vi "FGV Modbus.vi"(6 "Aktion":T1) -> (0 "error out":errorcluster)   [LabVIEW 2020, in "ABB-EL3000.lvlib" / "PMA.lvlib"]
uses:
  PMA.lvlib
  Allgemeine VI/Aktion FGV Modbus.ctl
  Aktion Adressen.ctl
  Allgemeine VI/Aktion Modbus lesen.ctl
  Aktion FGV Messwerte.ctl
  Allgemeine VI/Allgemeine VI.lvlib
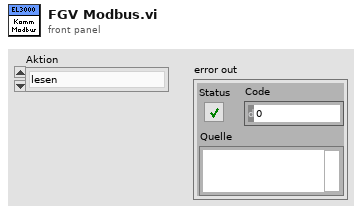
[diagram p1: front panel]
types:
  T1 = typedef "ABB-EL3000.lvlib/Allgemeine VI.lvlib/Aktion FGV Modbus.ctl" = enum16{"lesen", "Verbindung herstellen", "Verbindung trennen", "Komm", "Inaktiv"}
  T2 = typedef "ABB-EL3000.lvlib/PMA.lvlib/Aktion Adressen.ctl" = enum16{"lesen", "initialisieren"}
  T3 = typedef "ABB-EL3000.lvlib/PMA.lvlib/Aktion FGV Messwerte.ctl" = enum16{"lesen", "Messwerte", "Messbereich", "Status", "Diagnose Werte"}
  T4 = typedef "ABB-EL3000.lvlib/Allgemeine VI.lvlib/Aktion Modbus lesen.ctl" = enum16{"Coils", "Discrete Inputs", "Input Register", "Holding Register"}
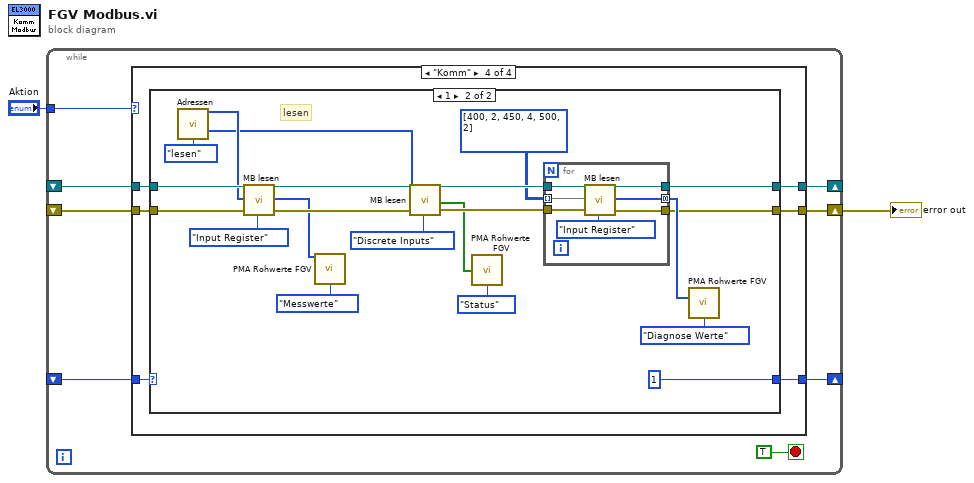
[diagram p0: block diagram]
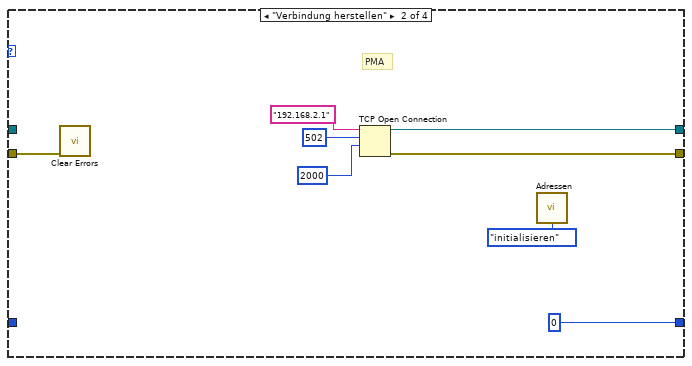
[diagram p3: hidden frame]
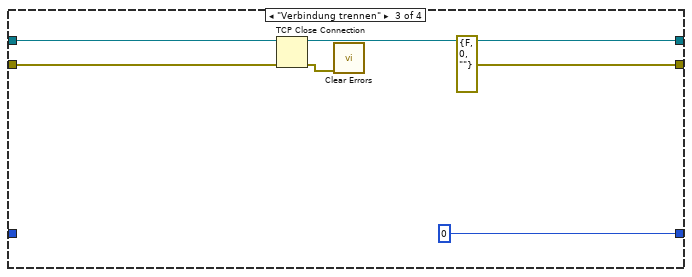
[diagram p4: hidden frame]
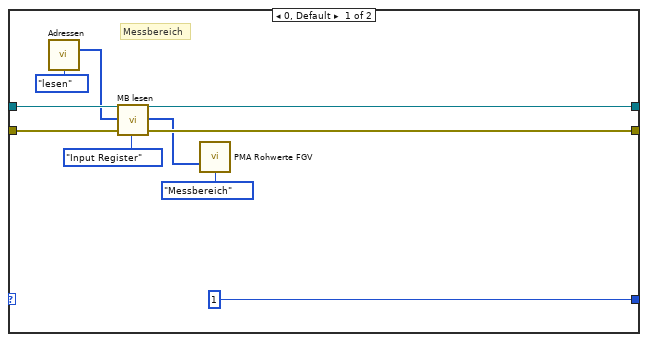
[diagram p5: hidden frame]
diagram:
  n1 = while {
    tunnel: "Aktion" -> [w9]
    shift-right: [w8] -> _
    shift-left: _ -> [w7]
    shift-right: [w6] -> w1
    shift-left: _ -> [w5]
    shift-right: [w3] -> _
    shift-left: _ -> [w4]
    stop <- TRUE stop-if-true
    n2 = case shown="\"Komm\"" w9 {
      tunnel: [w13 w20 w25 w32] -> w8
      tunnel: w7 -> [w13 _ w27 w33]
      tunnel: [w12 w19 errorcluster {"status"=FALSE, "code"=0, "source"=""} ("error out") w30] -> w6
      tunnel: w5 -> [w12 w18 w26 w31]
      tunnel: w4 -> [w11 _ _ w29]
      tunnel: [w11 0 0 w28] -> w3
      frame "lesen", Default {
      }
      frame "Verbindung herstellen" {
        # "PMA"
        n3 = call <vilib>:"Clear Errors.vi"("error in (no error)"=w18) -> ()  [unwired: 5 in, 2 out]
        n4 = TCP Open Connection(address="192.168.2.1" ("Adresse"), remote port or service name=u16 502 ("Netzwerk-Port oder -Dienst"), timeout ms (60000)=2000 ("Timeout in ms (60000)")) -> (connection ID=w20:refnum<k5>, error out=w19:errorcluster)  [unwired: 2 in]
        n5 = call "Adressen.vi"("Aktion"=Aktion_Adressen."initialisieren") -> ()  [unwired: 11 in, 4 out]
      }
      frame "Verbindung trennen" {
        n6 = TCP Close Connection(connection ID=w27, error in (no error)=w26) -> (connection ID out=w25:refnum<k5>, error out=w23:errorcluster)  [unwired: 1 in]
        n7 = call <vilib>:"Clear Errors.vi"("error in (no error)"=w23) -> ()  [unwired: 5 in, 2 out]
      }
      frame "Komm" {
        n8 = case shown="1" w29 {
          tunnel: w33 -> [w43 w64]
          tunnel: [w42 w45] -> w32
          tunnel: w31 -> [w41 w63]
          tunnel: [w40 w44] -> w30
          tunnel: [1 1] -> w28
          frame 0, Default {
            # "Messbereich"
            n9 = call "Adressen.vi"("Aktion"=Aktion_Adressen."lesen") -> ("Messbereich"=w36:u16[])  [unwired: 11 in, 3 out]
            n10 = call "MB lesen.vi"("TCP Refnum"=w43, "Adresse"=w36, "error in"=w41, "Aktion"=Aktion_Modbus_lesen."Input Register") -> ("TCP Refnum"=w42:refnum<k5>, "Input Registers"=w35:u16[], "error out"=w40:errorcluster)  [unwired: 17 in, 4 out]
            n11 = call "PMA Rohwerte FGV.vi"("Messbereich"=w35, "Aktion"=Aktion_FGV_Messwerte."Messbereich") -> ()  [unwired: 10 in, 4 out]
          }
          frame 1 {
            # "lesen"
            n12 = call "Adressen.vi"("Aktion"=Aktion_Adressen."lesen") -> ("Messwerte"=w61:u16[], "Gerätestatus"=w57:u16[])  [unwired: 11 in, 2 out]
            n13 = call "MB lesen.vi"("TCP Refnum"=w64, "Adresse"=w61, "error in"=w63, "Aktion"=Aktion_Modbus_lesen."Input Register") -> ("TCP Refnum"=w54:refnum<k5>, "Input Registers"=w52:u16[], "error out"=w55:errorcluster)  [unwired: 17 in, 4 out]
            n14 = call "PMA Rohwerte FGV.vi"("Messwerte"=w52, "Aktion"=Aktion_FGV_Messwerte."Messwerte") -> ()  [unwired: 10 in, 4 out]
            n15 = call "MB lesen.vi"("TCP Refnum"=w54, "Adresse"=w57, "error in"=w55, "Aktion"=Aktion_Modbus_lesen."Discrete Inputs") -> ("TCP Refnum"=w60:refnum<k5>, "Discrete Inputs"=w49:bool[], "error out"=w59:errorcluster)  [unwired: 17 in, 4 out]
            n16 = call "PMA Rohwerte FGV.vi"("Status"=w49, "Aktion"=Aktion_FGV_Messwerte."Status") -> ()  [unwired: 10 in, 4 out]
            n17 = for {
              tunnel: w60 -> [w71]
              tunnel: w59 -> [w70]
              tunnel: [w69] -> w44
              tunnel: [w68] -> w45
              tunnel: u16[][] [[400, 2], [450, 4], [500, 2]] ("Adresse") -> [w67] mode=indexing
              tunnel: [w65] -> w47 mode=concatenating
              n18 = call "MB lesen.vi"("TCP Refnum"=w71, "Adresse"=w67, "error in"=w70, "Aktion"=Aktion_Modbus_lesen."Input Register") -> ("TCP Refnum"=w68:refnum<k5>, "Input Registers"=w65:u16[], "error out"=w69:errorcluster)  [unwired: 17 in, 4 out]
            }
            n19 = call "PMA Rohwerte FGV.vi"("Diagnose Werte"=w47, "Aktion"=Aktion_FGV_Messwerte."Diagnose Werte") -> ()  [unwired: 10 in, 4 out]
          }
        }
      }
    }
  }
  "error out" <- w1
